vi "PreSpectraDe-meanAndHalveEnds.vi"(11 "Array":dbl[](array[numeric])) -> (0 "length":i32, 3 "PreppedArray":dbl[](array[numeric]))   [LabVIEW 2011]
doc: "Subtracts the mean from the signal, and halves the first and last values, Used prior to performing Power Spectrum.\nVI is configured \"Inline\", meaning it performs the same as if it was on its parent diagram."
uses:
  <vilib>/Analysis/NI_AALBase.lvlib
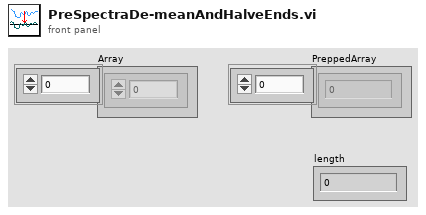
[diagram p1: front panel]
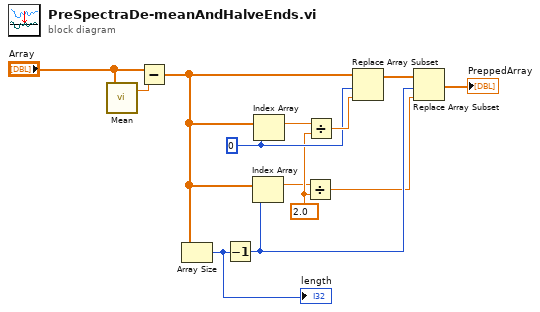
[diagram p0: block diagram]
diagram:
  w5 = 0
  w4 = 2.0
  n1 = call <vilib>:"Mean.vi"("X"="Array") -> ("mean"=w11:dbl)  [unwired: 1 out]
  n2 = Subtract(x="Array", y=w11) -> (x-y=w13:dbl[])
  n3 = Array Size(array=w13) -> (size(s)=w12:i32)
  "length" <- w12
  n4 = Decrement(x=w12) -> (x-1=w8:i32)
  n5 = Index Array(array=w13, index=w8) -> (element=w3:dbl)
  n6 = Index Array(array=w13, index=w5) -> (element=w2:dbl)
  n7 = Divide(x=w3, y=w4) -> (x/y=w7:dbl)
  n8 = Divide(x=w2, y=w4) -> (x/y=w6:dbl)
  n9 = Replace Array Subset(array=w13, new element=w6, index=w5) -> (w1:dbl[])
  n10 = Replace Array Subset(array=w1, new element=w7, index=w8) -> (→"PreppedArray":dbl[])
